vi "create.vi"(8 "error in (no error)":errorcluster, 11 "test in":refnum<class "test.lvclass">) -> (0 "error out":errorcluster, 3 "test out":refnum<class "test.lvclass">)   [LabVIEW 2018, in "test.lvclass"]
uses:
  test.lvclass
  TypeDef/Data.ctl
  test.lvclass/test.ctl
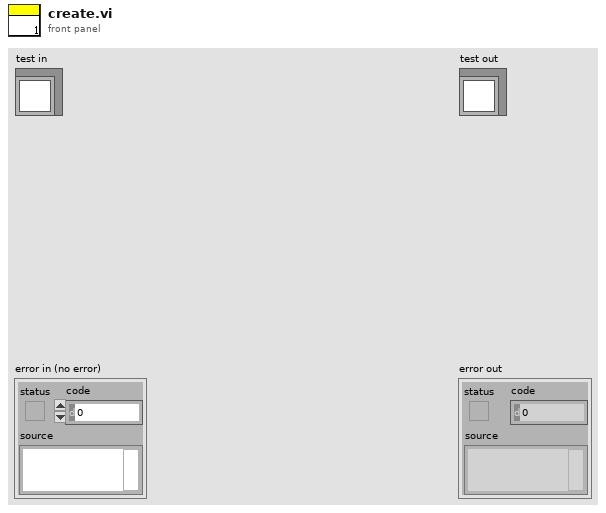
[diagram p1: front panel]
types:
  T1 = typedef "test.lvclass/Data.ctl" = cluster{"id":string, "config path":path, "value":i32, "flag":bool}
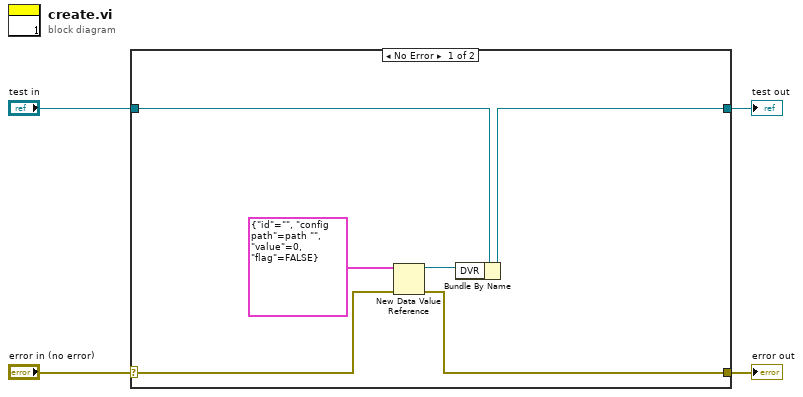
[diagram p0: block diagram]
diagram:
  n1 = case shown="No Error" "error in (no error)" {
    selector: "error in (no error)" -> [w7 w12]
    tunnel: [w6 w12] -> w3
    tunnel: [w8 w11] -> w1
    tunnel: "test in" -> [w10 w11]
    frame No Error {
      n2 = New Data Value Reference(data value=T1 {"id"="", "config path"=path "", "value"=0, "flag"=FALSE}, error in=w7) -> (data value reference=w5:refnum<data-value>, error out=w6:errorcluster)
      n3 = Bundle By Name(cluster=w10, "DVR"=w5) -> (w8:refnum<class "test.lvclass">)
    }
    frame Error {
    }
  }
  "error out" <- w3
  "test out" <- w1
